vi "Real-Time Main-testComm.vi"() -> ()   [LabVIEW 2016]
uses:
  <vilib>/userdefined/High Color/IMAQdx.ctl
  <vilib>/Platform/TimedLoop/XDataNode/timing_clust.ctl
  <vilib>/Platform/TimedLoop/XDataNode/nitl_modes.ctl
  <vilib>/Platform/TimedLoop/XDataNode/wakeup.ctl
  <vilib>/FPGAPlugInAG/roboRIO/niLvFpga_Open_roboRIO.vi
  <vilib>/rvi/interface/common/dynamic/niFpgaDynamicAddResources.vi
  <vilib>/FPGAPlugInAG/Dynamic/niLvFpga_Download_Dynamic.vi
  <vilib>/FPGAPlugInAG/Dynamic/niLvFpga_Run_Dynamic.vi
  <vilib>/Utility/error.llb/Error Cluster From Error Code.vi
  <vilib>/rvi/errors/niLvFpgaAdjustHostInterfaceError.vi
  <vilib>/Platform/TimedLoop/XDataNode/XDataNode.xnode
  <vilib>/rvi/interface/nirviOpenFPGA/nirviOpenFPGA.xnode
  FPGA Bitfiles/ImageProcessingw_FPGATarget_ImageProcessingw_Z23Lc7CsNwk.lvbitx
  <vilib>/rvi/interface/nirviMethod/nirviMethod.xnode
  <vilib>/rvi/interface/nirviReadWriteControl/nirviReadWriteControl.xnode
  <vilib>/Platform/TimedLoop/XDataNode/XDNodeRunTimeDep.lvlib
  <vilib>/vision/driver/NI_Vision_Acquisition_Software.lvlib
  <vilib>/rvi/interface/Simulation/niFpgaSimulationCallBeginRW.vi
  NiFpgaLv.dll
panel:
  out "Image Pixels (U32) 2":u32[][](array[numeric])
  out "# elements read":u32
  out "# elements write":u32
  out "Image Pixels (U32)":u32[](array[numeric])
  out "Image":T1(plugin-control)
  out "error out":errorcluster
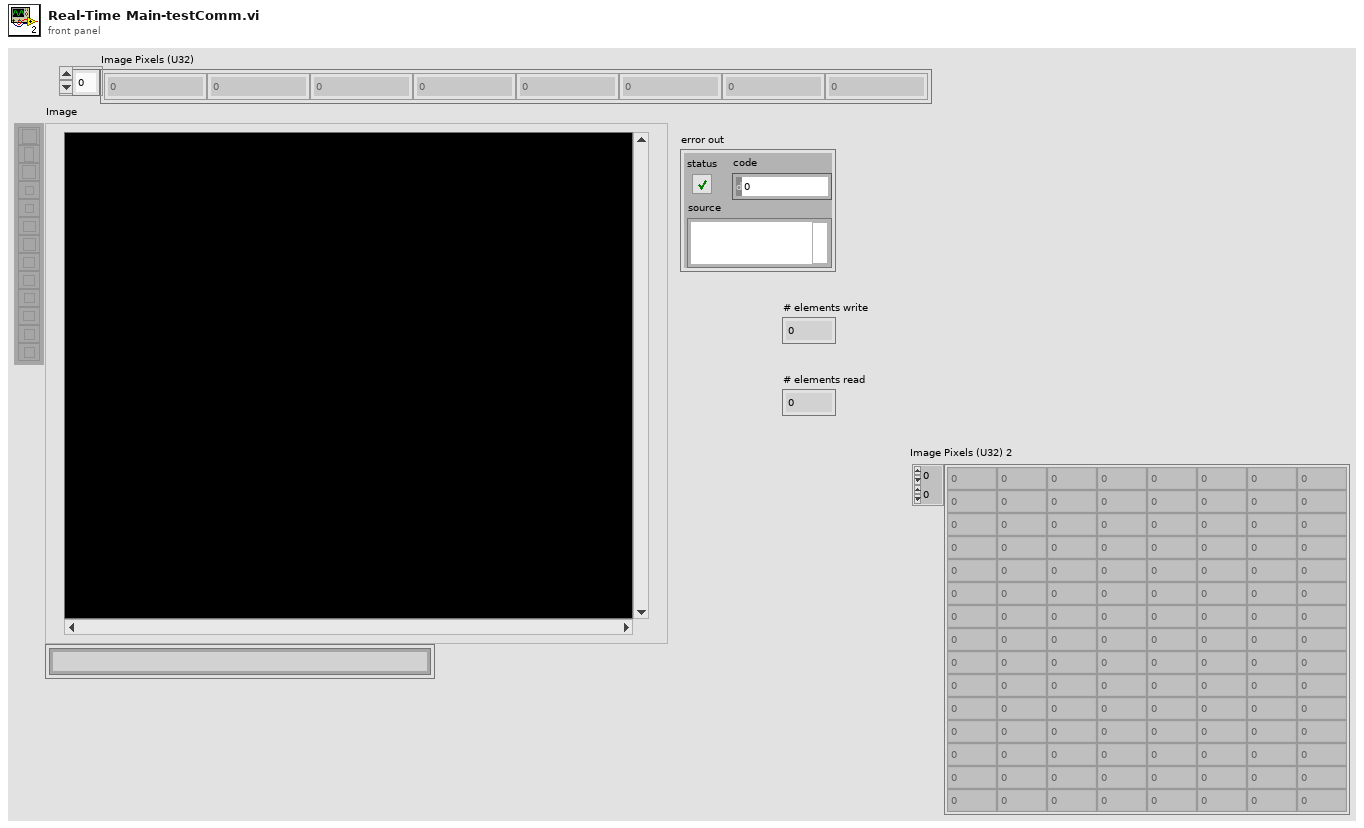
[diagram p1: front panel]
types:
  T1 = typedef "IMAQ Image.ctl" = refnum<image>
  T2 = typedef "Image Type" = u32
  T3 = typedef "IMAQdx.ctl" = refnum<k21>
  T4 = typedef "XDNodeRunTimeDep.lvlib/timing_clust.ctl" = cluster{"Expected End [f-1]":u64, "Actual End [f-1]":u64, "Finished Late? [f-1]":bool, "Expected End [i-1]":u64, "Actual End [i-1]":u64, "Finished Late? [i-1]":bool, "Expected Start [i]":u64, "Actual Start [i]":u64, "Expected Start [f]":u64, "Actual Start [f]":u64, "Source Name":string, "Structure Name":string, "Period":i64, "Deadline":i64, "Offset":i64, "Start":i64, "Priority":i32, "Timeout":i32, "Mode":T5, "Wakeup Reason":T6, "Error":errorcluster, "Source Type":string, "Secondary Source Type":string, "Global End Time":u64, "Global Start Time":u64, "Frame Duration":u64, "Iteration Duration":u64, "Assigned CPU":i32, "I/O Scan Engine Mode":u32}
  T5 = typedef "XDNodeRunTimeDep.lvlib/nitl_modes.ctl" = enum32{"No Change", "Process missed periods, maintain original phase", "Discard missed periods, maintain original phase", "Process missed periods, ignore original phase", "Discard missed periods, ignore original phase"}
  T6 = typedef "XDNodeRunTimeDep.lvlib/wakeup.ctl" = enum32{"Normal", "Aborted", "Asynchronous wakeup", "Timing source error", "Timed loop error", "Timeout"}
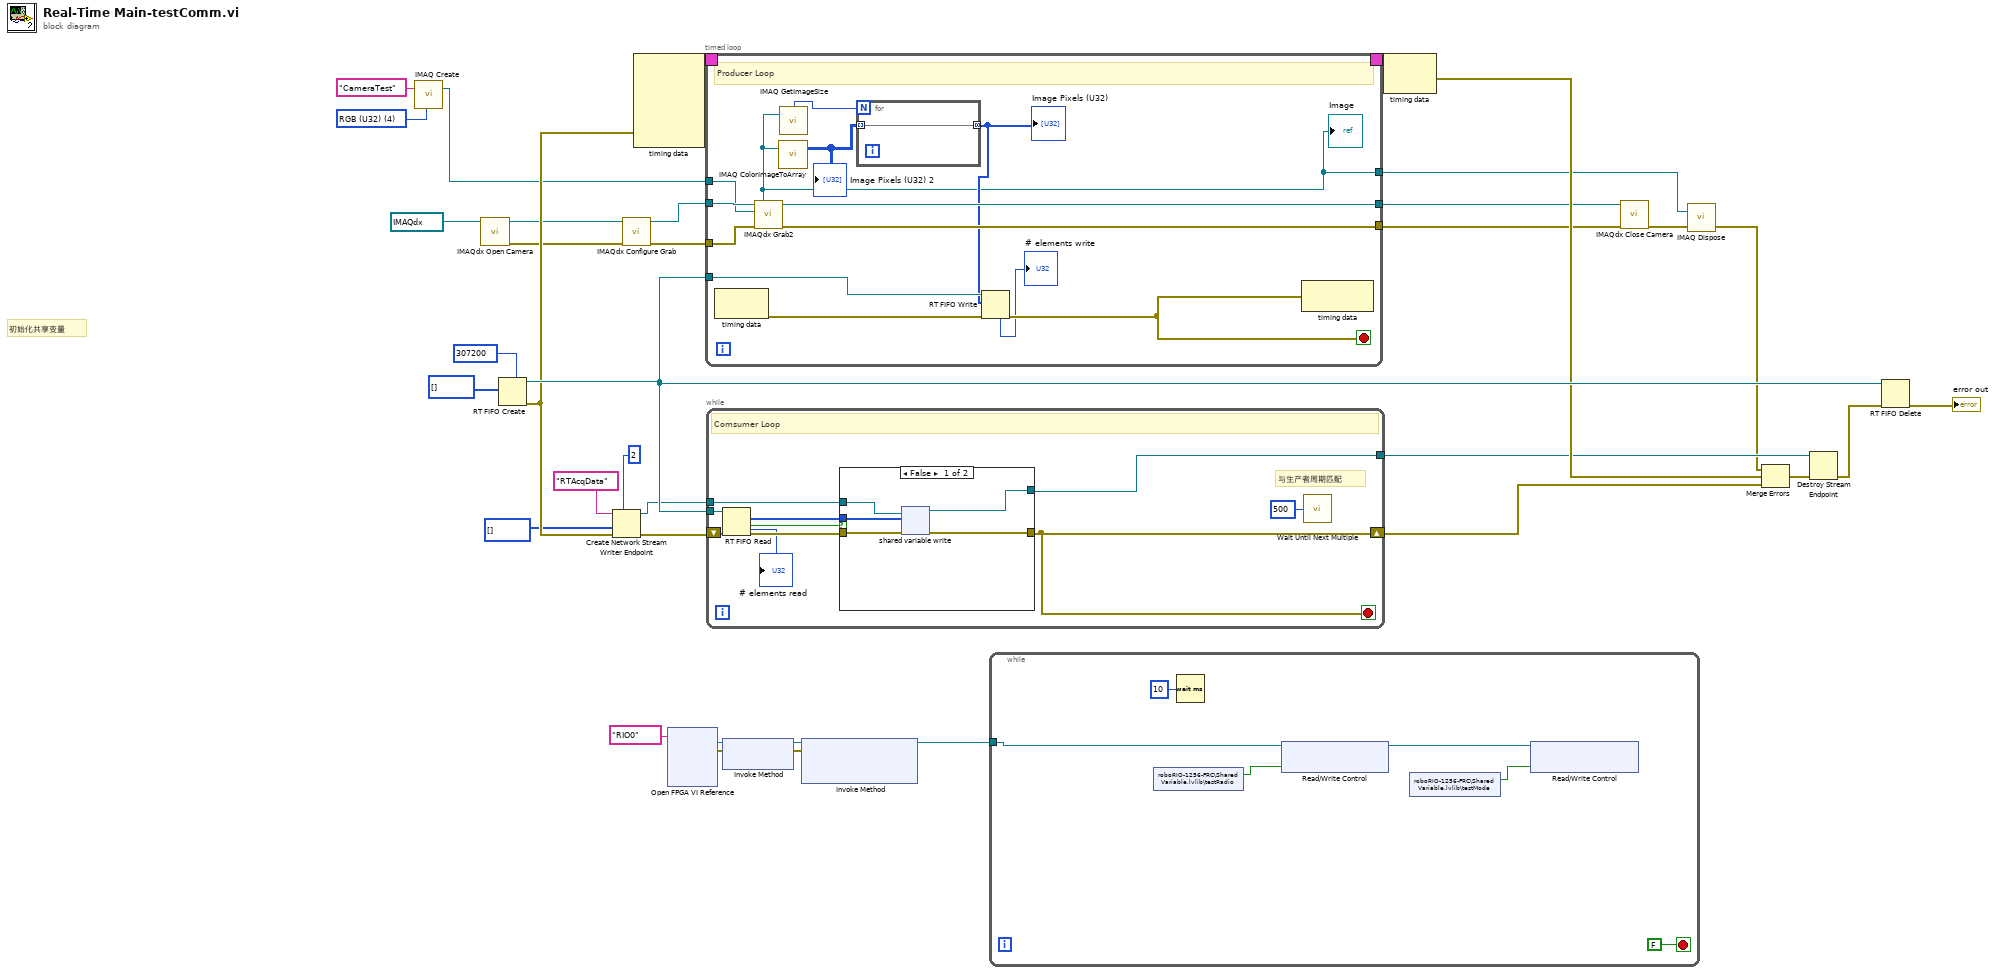
[diagram p0: block diagram]
diagram:
  w2 = T2 4 items=["Grayscale (U8)", "Grayscale (I16)", "Grayscale (SGL)", "Complex (CSG)", "RGB (U32)", "HSL (U32)", "RGB (U64)", "Grayscale (U16)"] ("Image Type")
  # "初始化共享变量"
  n1 = call "IMAQ Create"("Image Name"="CameraTest", "Image Type"=w2) -> ("New Image"=w3:T1)  [unwired: 3 in, 1 out]
  n2 = call <vilib>:"IMAQdx Open Camera.vi"("Session In"=T3 "cam0") -> ("error out"=w22:errorcluster, "Session Out"=w4:T3)  [unwired: 9 in]
  n3 = RT FIFO Create(1:i32[] [], 6:u32 307200 ("elements in array (1)")) -> (8:w33:refnum<k33>, 11:w28:errorcluster)  [unwired: 6 in, 1 out]
  n4 = Create Network Stream Writer Endpoint(7:2 ("writer buffer size"), 8:w28, 9:i32[] [], 11:"RTAcqData" ("writer name")) -> (0:w27:errorcluster, 3:w26:refnum<k21>)  [unwired: 3 in]
  n5 = call <vilib>:"IMAQdx Configure Grab.vi"("error in"=w22, "Session In"=w4) -> ("error out"=w21:errorcluster, "Session Out"=w20:T3)  [unwired: 8 in]
  n6 = node-c288(w28) -> (w36:T4)  [unwired: 4 in]
  n7 = xnode "Open FPGA VI Reference"("resource name"=tag "RIO0") -> ("FPGA VI Reference Out"=w5:refnum<k20>, "error out"=w6:errorcluster)  [unwired: 1 in]
  n8 = timed-loop {
    timing: w36 -> [_]
    timing-out: [_] -> w35
    tunnel: w33 -> [w47]
    tunnel: w21 -> [w46]
    tunnel: w20 -> [w45]
    tunnel: w3 -> [w44]
    tunnel: [w43] -> w19
    tunnel: [w38] -> w17
    tunnel: [w42] -> w16
    stop <- w48 stop-if-true
    # "Producer Loop"
    n9 = node-c288() -> (w49:errorcluster)  [unwired: 1 in]
    n10 = call <vilib>:"IMAQdx Grab2.vi"("error in"=w46, "Image In"=w44, "Session In"=w45) -> ("error out"=w42:errorcluster, "Image Out"=w38:T1, "Session Out"=w43:T3)  [unwired: 5 in, 1 out]
    "Image" <- w38
    n11 = call "IMAQ ColorImageToArray"("Image"=w38) -> ("Image Pixels (U32)"=w40:u32[][])  [unwired: 3 in, 2 out]
    "Image Pixels (U32) 2" <- w40
    n12 = call "IMAQ GetImageSize"("Image"=w38) -> ("X Resolution"=w41:i32)  [unwired: 3 in, 2 out]
    n13 = for {
      N: w41 -> [_]
      tunnel: w40 -> [w50] mode=indexing
      tunnel: [w50] -> w39 mode=concatenating
    }
    "Image Pixels (U32)" <- w39
    n14 = RT FIFO Write(0:w47, 1:w39, 3:w49) -> (7:→"# elements write":u32, 11:w48:errorcluster)  [unwired: 2 in, 2 out]
    n15 = node-c288(w48) -> ()  [unwired: 1 out]
  }
  n16 = while {
    tunnel: w33 -> [w64]
    shift-right: [w59] -> w31
    shift-left: w27 -> [w63]
    tunnel: w26 -> [w58]
    tunnel: [w57] -> w23
    stop <- w59 stop-if-true
    # "与生产者周期匹配"
    # "Comsumer Loop"
    n17 = RT FIFO Read(0:w64, 3:w63) -> (7:→"# elements read":u32, 9:w61:i32[], 10:w62:bool, 11:w60:errorcluster)  [unwired: 2 in, 1 out]
    n18 = case shown="False" w62 {
      tunnel: w61 -> [w66 _]
      tunnel: w60 -> [w69 w72]
      tunnel: [w68 w72] -> w59
      tunnel: w58 -> [w70 w71]
      tunnel: [w67 w71] -> w57
      frame False {
        n19 = shared-variable-write(w70, w69, w66) -> (w67:refnum<k21>, w68:errorcluster)  [unwired: 1 in, 1 out]
      }
      frame True {
      }
    }
    n20 = call "Wait Until Next Multiple"("Count(mSec)"=u32 500) -> ()  [unwired: 1 out]
  }
  n21 = xnode "Invoke Method"("FPGA VI Reference In"=w5, "error in"=w6) -> ("FPGA VI Reference Out"=w8:refnum<k20>, "error out"=w7:errorcluster)
  n22 = xnode "Invoke Method"("FPGA VI Reference In"=w8, "error in"=w7) -> ("FPGA VI Reference Out"=w1:refnum<k20>)  [unwired: 1 in, 1 out]
  n23 = while {
    tunnel: w1 -> [w78]
    stop <- FALSE stop-if-true
    n24 = shared-variable "roboRIO-1256-FRC\\Shared Variable.lvlib\\testRadio"() -> (w73:bool)  [unwired: 1 in, 1 out]
    n25 = Wait (ms)(milliseconds to wait=u32 10) -> ()  [unwired: 1 out]
    n26 = xnode "Read/Write Control"("FPGA VI Reference In"=w78, "Radio LED Status"=w73) -> ("FPGA VI Reference Out"=w77:refnum<k20>)  [unwired: 1 in, 1 out]
    n27 = shared-variable "roboRIO-1256-FRC\\Shared Variable.lvlib\\testMode"() -> (w74:bool)  [unwired: 1 in, 1 out]
    n28 = xnode "Read/Write Control"("FPGA VI Reference In"=w77, "Mode LED Status"=w74) -> ()  [unwired: 1 in, 2 out]
  }
  n29 = node-c288(w35) -> (w32:errorcluster)
  n30 = call <vilib>:"IMAQdx Close Camera.vi"("error in"=w16, "Session In"=w19) -> ("error out"=w18:errorcluster)  [unwired: 9 in]
  n31 = call "IMAQ Dispose"("Image"=w17, "error in (no error)"=w18) -> ("error out"=w15:errorcluster)  [unwired: 4 in]
  n32 = Merge Errors(w15, w32, w31) -> (w25:errorcluster)
  n33 = Destroy Stream Endpoint(8:w25, 11:w23) -> (0:w24:errorcluster)
  n34 = RT FIFO Delete(0:w33, 3:w24) -> (11:→"error out":errorcluster)  [unwired: 1 in]
